vi "HP34970A Conf Trigger.vi"(0 "VISA session":refnum<visa-resource-name>, 1 "Set/Check (F:Set)":bool, 2 "Check Parameter(0:Source)":T3(ring), 3 "Wait for Trigger? (F:No)":bool, 5 "Source (1:Immediate)":T2(ring)=enum."Immediate", 7 "Scan-Scan Interval (1:Min)":enum16{"Manual", "Minimum", "Maximum"}(ring)=enum."Minimum", 9 "Interval Value (0)":dbl min=0.0 max=359999.0 format="%.2f", 11 "error in (no error)":errorcluster, 12 "Max Trigger Count (3:Inf)":T1(ring)=enum."Infinity", 13 "# Triggers (1)":u16=1 min=1 max=50000 step=1) -> (4 "dup VISA session":refnum<visa-resource-name>, 8 "Configuration ?":string, 15 "error out":errorcluster)   [LabVIEW 2020]
doc: "This VI lets you configure the instrument's triggering parameters. For example, you can set the trigger source, scan interval, etc.\n\nAfter configuration, you can put the instrument into \"wait for trigger\" mode."
panel:
  # "Check\nSet"
  # "Yes\nNo"
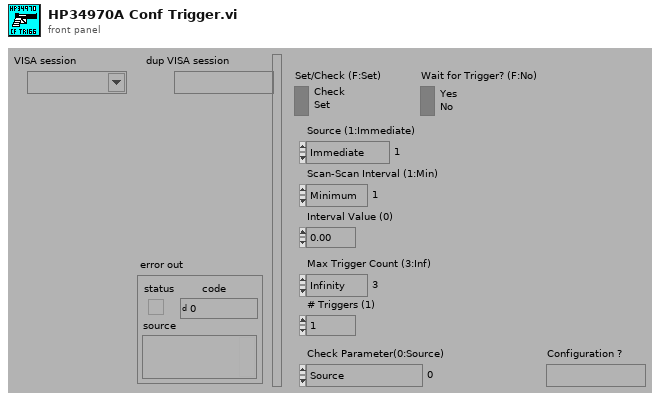
[diagram p1: front panel]
types:
  T1 = enum16{"Manual", "Minimum", "Maximum", "Infinity"}
  T2 = enum16{"Bus", "Immediate", "External", "Alarm 1", "Alarm 2", "Alarm 3", "Alarm 4", "Timer"}
  T3 = enum16{"Source", "Scan-Scan Interval", "Max Trigger Count"}
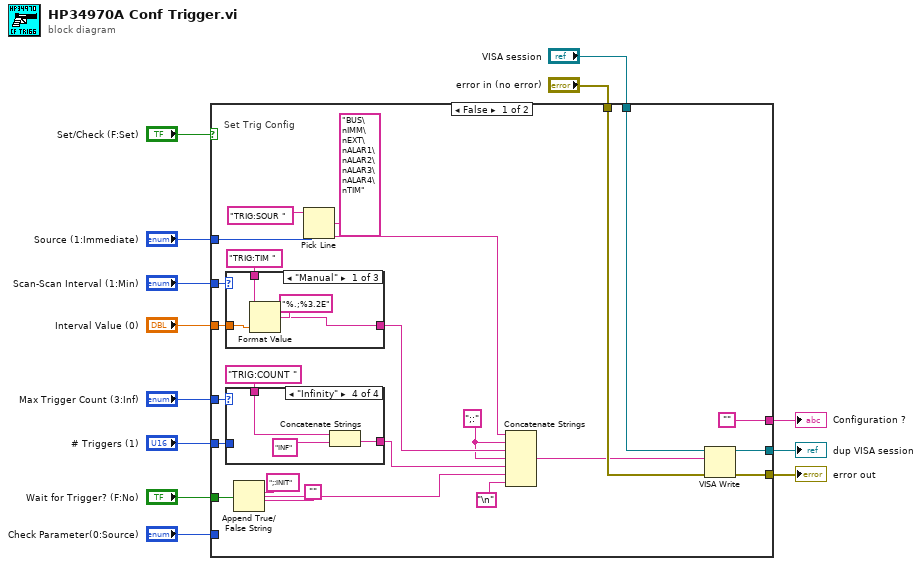
[diagram p0: block diagram]
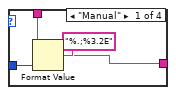
[diagram p2: hidden frame]
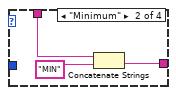
[diagram p3: hidden frame]
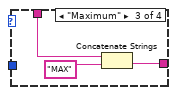
[diagram p4: hidden frame]
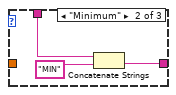
[diagram p5: hidden frame]
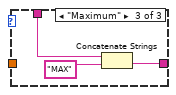
[diagram p6: hidden frame]
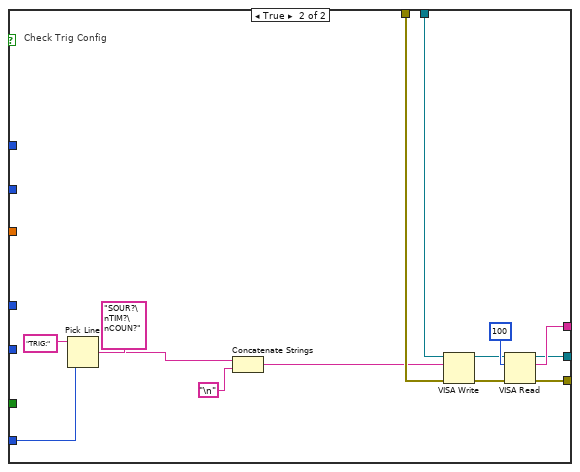
[diagram p7: hidden frame]
diagram:
  n1 = case shown="False" "Set/Check (F:Set)" {
    tunnel: [w33 w74] -> w12
    tunnel: [w34 w71] -> w13
    tunnel: ["" w72] -> w10
    tunnel: "VISA session" -> [w36 w70]
    tunnel: "error in (no error)" -> [w35 w69]
    tunnel: "Check Parameter(0:Source)" -> [_ w64]
    tunnel: "Source (1:Immediate)" -> [w30 _]
    tunnel: "Scan-Scan Interval (1:Min)" -> [w29 _]
    tunnel: "Interval Value (0)" -> [w27 _]
    tunnel: "Max Trigger Count (3:Inf)" -> [w25 _]
    tunnel: "# Triggers (1)" -> [w24 _]
    tunnel: "Wait for Trigger? (F:No)" -> [w16 _]
    frame False {
      w21 = ";:"
      # "Set Trig Config"
      n2 = case shown="\"Manual\"" w29 {
        tunnel: "TRIG:TIM " -> [w53 w57 w59]
        tunnel: w27 -> [w52 _ _]
        tunnel: [w51 w55 w58] -> w22
        frame "Manual" {
          n3 = Format Value(string ("")=w53, format string="%.;%3.2E", value (0)=w52) -> (output string=w51:string)
        }
        frame "Minimum" {
          n4 = Concatenate Strings(w57, "MIN") -> (w55:string)
        }
        frame "Maximum" {
          n5 = Concatenate Strings(w59, "MAX") -> (w58:string)
        }
      }
      n6 = case shown="\"Infinity\"" w25 {
        tunnel: "TRIG:COUNT " -> [w40 w44 w46 w49]
        tunnel: [w39 w42 w45 w48] -> w20
        tunnel: w24 -> [w38 _ _ _]
        frame "Manual" {
          n7 = Format Value(string ("")=w40, format string="%.;%3.2E", value (0)=w38) -> (output string=w39:string)
        }
        frame "Minimum" {
          n8 = Concatenate Strings(w44, "MIN") -> (w42:string)
        }
        frame "Maximum" {
          n9 = Concatenate Strings(w46, "MAX") -> (w45:string)
        }
        frame "Infinity" {
          n10 = Concatenate Strings(w49, "INF") -> (w48:string)
        }
      }
      n11 = Append True/False String(1:w16, 2:"", 3:";:INIT" ("true string")) -> (0:w15:string)  [unwired: 1 in]
      n12 = Pick Line(string ("")="TRIG:SOUR ", multi-line string="BUS\nIMM\nEXT\nALAR1\nALAR2\nALAR3\nALAR4\nTIM", line index=w30) -> (output string=w23:string)
      n13 = Concatenate Strings(w23, w21, w22, w21, w20, w15, "\n") -> (w19:string)
      n14 = VISA Write(VISA resource name=w36, write buffer=w19, error in (no error)=w35) -> (VISA resource name out=w34:refnum<visa-resource-name>, error out=w33:errorcluster)  [unwired: 1 out]
    }
    frame True {
      # "Check Trig Config"
      n15 = Pick Line(string ("")="TRIG:", multi-line string="SOUR?\nTIM?\nCOUN?", line index=w64) -> (output string=w62:string)
      n16 = Concatenate Strings(w62, "\n") -> (w61:string)
      n17 = VISA Write(VISA resource name=w70, write buffer=w61, error in (no error)=w69) -> (VISA resource name out=w68:refnum<visa-resource-name>, error out=w67:errorcluster)  [unwired: 1 out]
      n18 = VISA Read(VISA resource name=w68, byte count=u32 100 ("byte count (0)"), error in (no error)=w67) -> (VISA resource name out=w71:refnum<visa-resource-name>, read buffer=w72:string, error out=w74:errorcluster)  [unwired: 1 out]
    }
  }
  "dup VISA session" <- w13
  "error out" <- w12
  "Configuration ?" <- w10
